vi "myRIO_BRig_RT__Case_Exp_State_Cue1__v4.vi"(0 "input_state":T1, 1 "input_dataCurrent":u16[](array[numeric]), 6 "I_lick":bool, 7 "input_arrTrig":bool[](array[boolean])) -> (12 "output_SelectionState":bool, 13 "output_CueLed_Event":bool, 14 "output_state":T1, 15 "output_dataCurrent":u16[](array[numeric]), 16 "output_l1_laserEvent":bool, 17 "output_l1_laserOn":bool, 18 "output_l2_laserEvent":bool, 19 "output_l2_laserOn":bool)   [LabVIEW 2014]
uses:
  myRIO_BRig_RT__Case_Exp_stateList.ctl
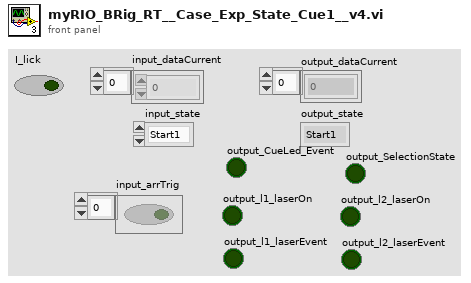
[diagram p1: front panel]
types:
  T1 = typedef "myRIO_BRig_RT__Case_Exp_stateList.ctl" = enum16{"Start1", "Start2", "Start3", "saveSettings1", "saveSettings2", "saveSettings3", "saveSettings4", "saveSettings_LC_ENL_l1", "saveSettings_LC_ENL_l2", "saveSettings_LC_Cue_l1", "saveSettings_LC_Cue_l2", "saveSettings6_LC_l1_Other", "SaveSettings6_LC_l2_Other", "setSettings_Audio", "setSettings_Laser", "initBlock_pre", "initBlock", "initBlock2", "initBlock_post", "initTrial_pre", "initTrial", "initTrial2", "initTrial3", "initTrial4", "initTrial_LC_ENL1", "initTrial_LC_Cue1", "initTrial_LC_Cue1_2", "initTrial_LC_Sel", "initTrial_post", "ENL1_pre", "ENL1", "ENL1_post", "ENL1Penalty_pre", "ENL1Penalty", "ENL2_pre", "ENL2", "ENL2Penalty_pre", "ENL2Penalty", "Cue1_pre", "Cue1", "Cue1_post", "Cue1Penalty_pre", "Cue1Penalty", "Cue2_pre", "Cue2", "Cue2Penalty_pre", "Cue2Penalty", "Selection_pre", "Selection", "Select_post", "SelectReward_pre", "SelectReward", "SelectRewardPost_pre", "SelectRewardPost", "SelectWrong_pre", "SelectWrong", "SelectWrong_post", "SelectTimeout_pre", "SelectTimeout", "SelectTimeout_post", "endTrial_pre", "endTrial1", "endTrial2", "endTrial3", "endTrial_post", "endBlock_pre", "endBlock", "endBlock_post", "endExp", "commConnect", "commUpload_pre", "commUpload_dataBlock", "commUpload_dataCurrent", "commUpload_dataExp", "commUpload_dataLC", "commUpload_dataTrial", "commUpload_post", "saveData_pre", "saveData_dataBlock", "saveData_dataCurrent", "saveData_dataExp", "saveData_dataLC", "saveData_dataTrial", "saveData_post", "empty_endBlock1", "empty_endBlock2", "empty_endTrial1", "empty_endTrial2", "empty_endTrial3", "empty_endTrial4", "empty_endTrial5", "dummyState", "dummyState_endBlock"}
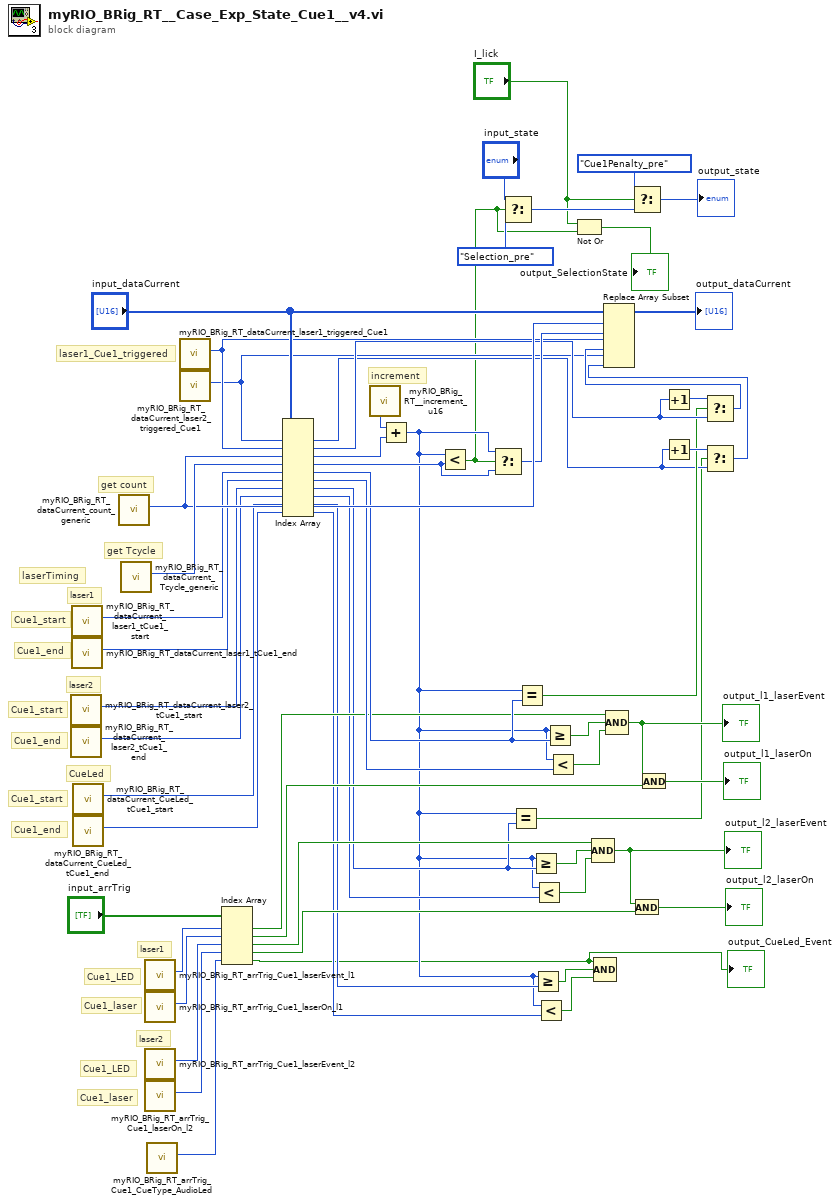
[diagram p0: block diagram]
diagram:
  # "Cue1_end"
  # "Cue1_start"
  # "CueLed"
  # "Cue1_LED"
  # "Cue1_laser"
  # "Cue1_LED"
  # "Cue1_laser"
  # "laser2"
  # "laser1"
  # "Cue1_end"
  # "Cue1_start"
  # "laser2"
  # "laser1"
  # "Cue1_end"
  # "Cue1_start"
  # "laser1_Cue1_triggered"
  # "laserTiming"
  # "increment"
  # "get Tcycle"
  # "get count"
  n1 = call "myRIO_BRig_RT_dataCurrent_laser2_tCue1_start.vi"() -> ("output_laser2_tCue1_start"=w35:i32)  [unwired: 11 in]
  n2 = call "myRIO_BRig_RT_dataCurrent_laser2_tCue1_end.vi"() -> ("output_laser2_tCue1_end"=w34:i32)  [unwired: 11 in]
  n3 = call "myRIO_BRig_RT_dataCurrent_laser1_tCue1_start.vi"() -> ("output_laser1_tCue1_start"=w37:i32)  [unwired: 11 in]
  n4 = call "myRIO_BRig_RT_dataCurrent_laser1_tCue1_end.vi"() -> ("output_laser1_tCue1_end"=w36:i32)  [unwired: 11 in]
  n5 = call "myRIO_BRig_RT_dataCurrent_CueLed_tCue1_start.vi"() -> ("output_CueLed_tCue1_start"=w19:i32)  [unwired: 11 in]
  n6 = call "myRIO_BRig_RT_dataCurrent_CueLed_tCue1_end.vi"() -> ("output_CueLed_tCue1_end"=w18:i32)  [unwired: 11 in]
  n7 = call "myRIO_BRig_RT_dataCurrent_count_generic.vi"() -> ("output_count_generic"=w57:i32)  [unwired: 11 in]
  n8 = call "myRIO_BRig_RT_dataCurrent_Tcycle_generic.vi"() -> ("output_Tcycle_generic"=w58:i32)  [unwired: 11 in]
  n9 = call "myRIO_BRig_RT_arrTrig_Cue1_laserEvent_l1.vi"() -> ("output_arrTrig_Cue1_laserEvent_l1"=w32:i32)  [unwired: 11 in]
  n10 = call "myRIO_BRig_RT_arrTrig_Cue1_laserOn_l1.vi"() -> ("output_arrTrig_Cue1_laserOn_l1"=w31:i32)  [unwired: 11 in]
  n11 = call "myRIO_BRig_RT_arrTrig_Cue1_laserEvent_l2.vi"() -> ("output_arrTrig_Cue1_laserEvent_l2"=w30:i32)  [unwired: 11 in]
  n12 = call "myRIO_BRig_RT_arrTrig_Cue1_laserOn_l2.vi"() -> ("output_arrTrig_Cue1_laserOn_l2"=w29:i32)  [unwired: 11 in]
  n13 = call "myRIO_BRig_RT_arrTrig_Cue1_CueType_AudioLed.vi"() -> ("output_arrTrig_Cue1_CueType_AudioLed"=w13:i32)  [unwired: 11 in]
  n14 = call "myRIO_BRig_RT_dataCurrent_laser1_triggered_Cue1.vi"() -> ("output_laser1_triggered_Cue1"=w43:i32)  [unwired: 11 in]
  n15 = call "myRIO_BRig_RT_dataCurrent_laser2_triggered_Cue1.vi"() -> ("output_laser2_triggered_Cue1"=w12:i32)  [unwired: 11 in]
  n16 = Index Array(array="input_arrTrig", index #1=w32, index #2=w31, index #3=w30, index #4=w29, index #5=w13) -> (element #1=w27:bool, element #2=w28:bool, element #3=w26:bool, element #4=w25:bool, element #5=w4:bool)
  "output_CueLed_Event" <- w4
  n17 = Index Array(array="input_dataCurrent", index #1=w12, index #2=w43, index #3=w57, index #4=w58, index #5=w37, index #6=w36, index #7=w35, index #8=w34, index #9=w19, index #10=w18) -> (element #1=w9:u16, element #2=w41:u16, element #3=w39:u16, element #4=w56:u16, element #5=w38:u16, element #6=w45:u16, element #7=w7:u16, element #8=w24:u16, element #9=w17:u16, element #10=w16:u16)
  n18 = call "myRIO_BRig_RT__increment_u16.vi"() -> ("output_increment__u16"=w53:u16)  [unwired: 11 in]
  n19 = Add(x=w53, y=w39) -> (x+y=w6:u16)
  n20 = Less?(x=w6, y=w56) -> (x < y?=w2:bool)
  n21 = Select(t=w6, s=w2, f=w56) -> (s? t:f=w55:u16)
  n22 = Select(t="input_state", s=w2, f=myRIO_BRig_RT__Case_Exp_stateList."Selection_pre" ("Enum")) -> (s? t:f=w54:T1)
  n23 = Equal?(x=w6, y=w7) -> (x = y?=w5:bool)
  n24 = Equal?(x=w6, y=w38) -> (x = y?=w10:bool)
  n25 = Greater Or Equal?(x=w6, y=w7) -> (x >= y?=w23:bool)
  n26 = Greater Or Equal?(x=w6, y=w17) -> (x >= y?=w15:bool)
  n27 = Less?(x=w6, y=w24) -> (x < y?=w22:bool)
  n28 = Less?(x=w6, y=w16) -> (x < y?=w14:bool)
  n29 = Greater Or Equal?(x=w6, y=w38) -> (x >= y?=w51:bool)
  n30 = Less?(x=w6, y=w45) -> (x < y?=w52:bool)
  n31 = Not Or(1:w2, 2:"I_lick") -> (0:→"output_SelectionState":bool)
  n32 = Compound Arithmetic op=AND(w26, w23, w22) -> (w21:bool)
  "output_l2_laserEvent" <- w21
  n33 = Compound Arithmetic op=AND(w4, w15, w14) -> ()  [unwired: 1 out]
  n34 = Compound Arithmetic op=AND(w27, w51, w52) -> (w40:bool)
  "output_l1_laserEvent" <- w40
  n35 = Select(t=myRIO_BRig_RT__Case_Exp_stateList."Cue1Penalty_pre" ("Enum"), s="I_lick", f=w54) -> (s? t:f=→"output_state":T1)
  n36 = And(x=w21, y=w25) -> (x .and. y?=→"output_l2_laserOn":bool)
  n37 = And(x=w40, y=w28) -> (x .and. y?=→"output_l1_laserOn":bool)
  n38 = Increment(x=w41) -> (x+1=w42:u16)
  n39 = Increment(x=w9) -> (x+1=w11:u16)
  n40 = Select(t=w42, s=w10, f=w41) -> (s? t:f=w44:u16)
  n41 = Select(t=w11, s=w5, f=w9) -> (s? t:f=w8:u16)
  n42 = Replace Array Subset(array="input_dataCurrent", new element #1=w55, index #1=w57, new element #2=w44, index #2=w43, new element #3=w8, index #3=w12) -> (→"output_dataCurrent":u16[])
